vi "Delete.vi"(8 "error in (no error)":errorcluster, 11 "IAmGLF in":refnum<class "IAmGLF.lvclass">) -> (0 "error out":errorcluster)   [LabVIEW 2024, in "GLF.lvlib" / "IAmGLF.lvclass"]
uses:
  IAmGLF.lvclass
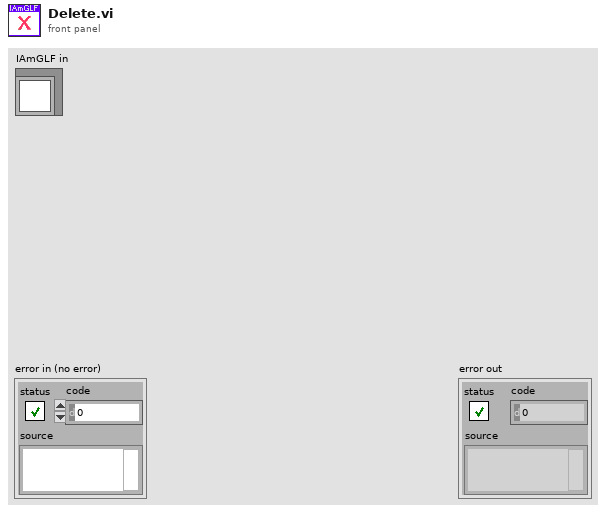
[diagram p1: front panel]
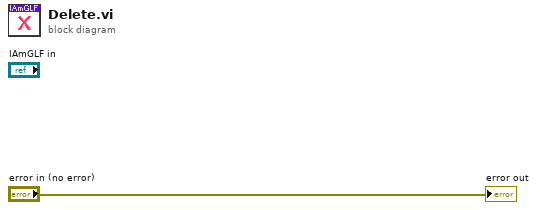
[diagram p0: block diagram]
diagram:
  "error out" <- "error in (no error)"
